vi "Interfaz_Computador.vi"() -> ()   [LabVIEW 2014]
uses:
  <vilib>/lvdsc/process/Deploy Library.vi
  <vilib>/lvdsc/process/Undeploy Library.vi
  <vilib>/lvdsc/NI_DSC.lvlib
panel:
  out "output cluster":T1
  out "error out":errorcluster
  in  "stop":bool
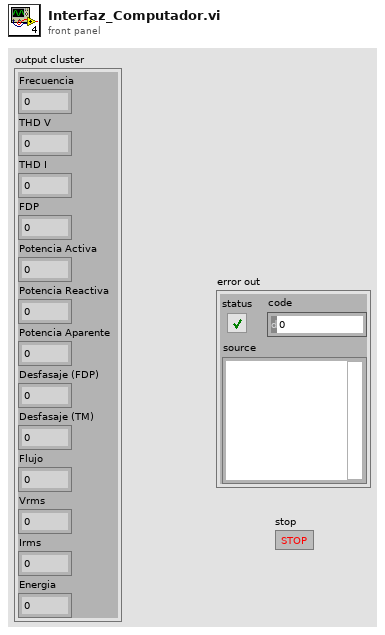
[diagram p1: front panel]
types:
  T1 = cluster{"Frecuencia":dbl, "THD V":dbl, "THD I":dbl, "FDP":dbl, "Potencia Activa":dbl, "Potencia Reactiva":dbl, "Potencia Aparente":dbl, "Desfasaje (FDP)":dbl, "Desfasaje (TM)":dbl, "Flujo":dbl, "Vrms":dbl, "Irms":dbl, "Energia":dbl}
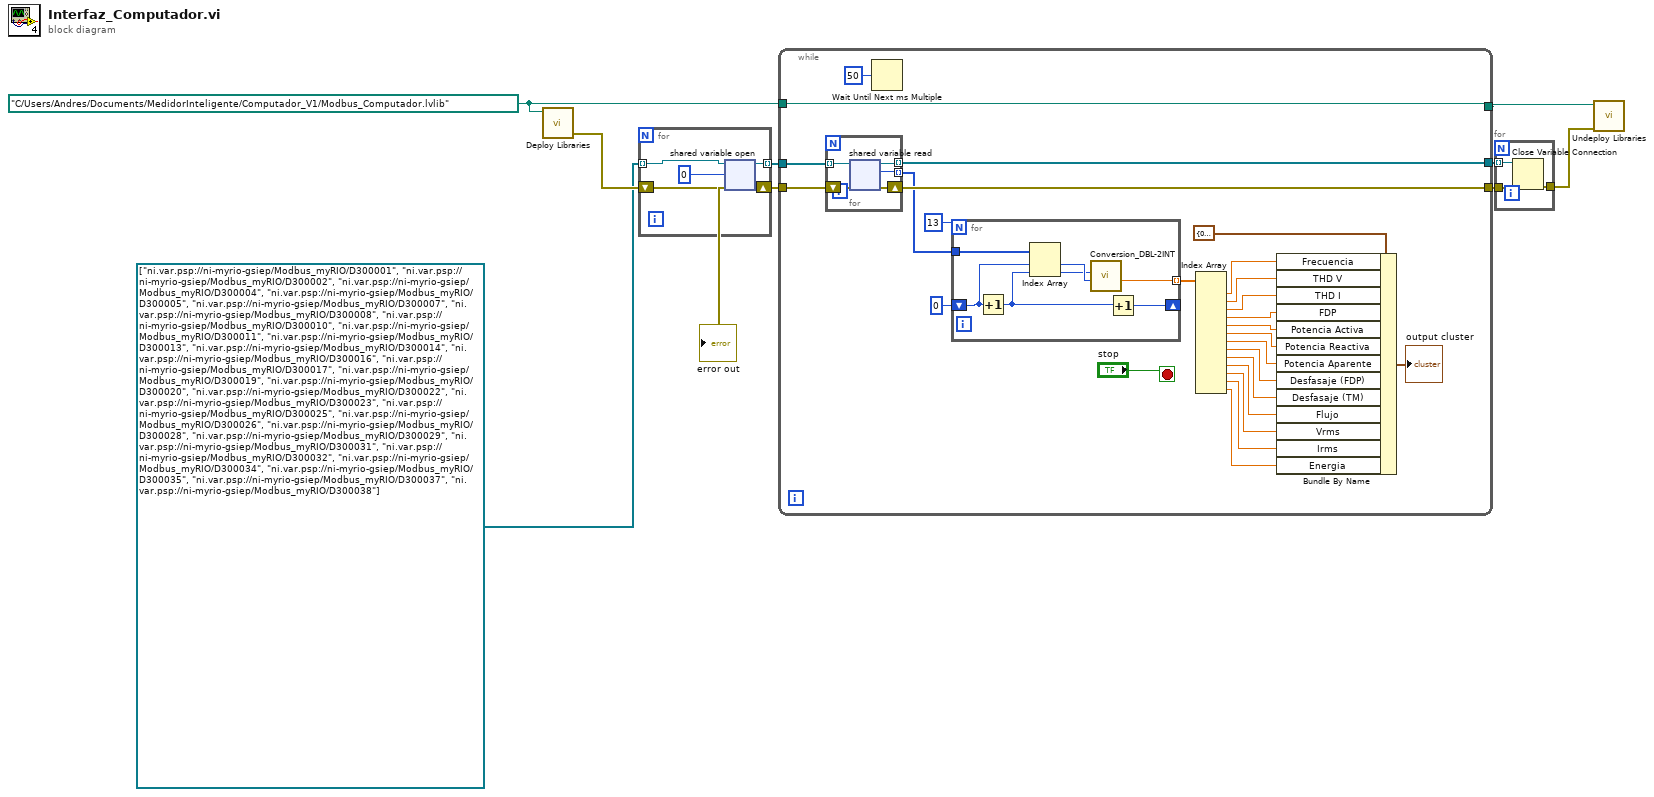
[diagram p0: block diagram]
diagram:
  w7 = path "C:/Users/Andres/Documents/MedidorInteligente/Computador_V1/Modbus_Computador.lvlib" ("library path")
  n1 = call-poly <vilib>:"Deploy Libraries.vi"("library path"=w7) -> ("error out"=w9:errorcluster)  [unwired: 8 in]
  n2 = for {
    tunnel: refnum<k21>[] ["ni.var.psp://ni-myrio-gsiep/Modbus_myRIO/D300001", "ni.var.psp://ni-myrio-gsiep/Modbus_myRIO/D300002", "ni.var.psp://ni-myrio-gsiep/Modbus_myRIO/D300004", "ni.var.psp://ni-myrio-gsiep/Modbus_myRIO/D300005", "ni.var.psp://ni-myrio-gsiep/Modbus_myRIO/D300007", "ni.var.psp://ni-myrio-gsiep/Modbus_myRIO/D300008", "ni.var.psp://ni-myrio-gsiep/Modbus_myRIO/D300010", "ni.var.psp://ni-myrio-gsiep/Modbus_myRIO/D300011", "ni.var.psp://ni-myrio-gsiep/Modbus_myRIO/D300013", "ni.var.psp://ni-myrio-gsiep/Modbus_myRIO/D300014", "ni.var.psp://ni-myrio-gsiep/Modbus_myRIO/D300016", "ni.var.psp://ni-myrio-gsiep/Modbus_myRIO/D300017", "ni.var.psp://ni-myrio-gsiep/Modbus_myRIO/D300019", "ni.var.psp://ni-myrio-gsiep/Modbus_myRIO/D300020", "ni.var.psp://ni-myrio-gsiep/Modbus_myRIO/D300022", "ni.var.psp://ni-myrio-gsiep/Modbus_myRIO/D300023", "ni.var.psp://ni-myrio-gsiep/Modbus_myRIO/D300025", "ni.var.psp://ni-myrio-gsiep/Modbus_myRIO/D300026", "ni.var.psp://ni-myrio-gsiep/Modbus_myRIO/D300028", "ni.var.psp://ni-myrio-gsiep/Modbus_myRIO/D300029", "ni.var.psp://ni-myrio-gsiep/Modbus_myRIO/D300031", "ni.var.psp://ni-myrio-gsiep/Modbus_myRIO/D300032", "ni.var.psp://ni-myrio-gsiep/Modbus_myRIO/D300034", "ni.var.psp://ni-myrio-gsiep/Modbus_myRIO/D300035", "ni.var.psp://ni-myrio-gsiep/Modbus_myRIO/D300037", "ni.var.psp://ni-myrio-gsiep/Modbus_myRIO/D300038"] -> [w10] mode=indexing
    shift-right: [w13] -> w8
    shift-left: w9 -> [w14]
    tunnel: [w12] -> w6 mode=indexing
    n3 = shared-variable-open(w10, w14, u32 0) -> (w12:refnum<k21>, w13:errorcluster)  [unwired: 1 in]
  }
  "error out" <- w8
  n4 = while {
    tunnel: w8 -> [w40]
    tunnel: [w39] -> w4
    tunnel: [w38] -> w5
    tunnel: w7 -> [w38]
    tunnel: w6 -> [w36]
    tunnel: [w34] -> w3
    stop <- "stop" stop-if-true
    n5 = for {
      tunnel: w36 -> [w50] mode=indexing
      shift-right: [w51] -> w39
      shift-left: w40 -> [w52]
      tunnel: [w49] -> w34 mode=indexing
      tunnel: [w48] -> w33 mode=indexing
      n6 = shared-variable-read(w50, w52) -> (w49:refnum<k21>, w51:errorcluster, w48:u32)  [unwired: 1 out]
    }
    n7 = Wait Until Next ms Multiple(millisecond multiple=u32 50) -> ()  [unwired: 1 out]
    n8 = for {
      N: 13 -> [_]
      tunnel: w33 -> [w47]
      shift-right: [w44] -> _
      shift-left: 0 -> [w46]
      tunnel: [w43] -> w29 mode=indexing
      n9 = Increment(x=w46) -> (x+1=w45:i32)
      n10 = Index Array(array=w47, index #1=w46, index #2=w45) -> (element #1=w42:u32, element #2=w41:u32)
      n11 = call "Conversion_DBL-2INT.vi"("Integer LOW"=w42, "Integer HIGH"=w41) -> ("Double"=w43:dbl)  [unwired: 2 in, 3 out]
      n12 = Increment(x=w45) -> (x+1=w44:i32)
    }
    n13 = Index Array(array=w29) -> (element #1=w28:dbl, element #2=w27:dbl, element #3=w26:dbl, element #4=w25:dbl, element #5=w24:dbl, element #6=w23:dbl, element #7=w22:dbl, element #8=w21:dbl, element #9=w20:dbl, element #10=w19:dbl, element #11=w18:dbl, element #12=w17:dbl, element #13=w16:dbl)  [unwired: 13 in]
    n14 = Bundle By Name(cluster=T1 {"Frecuencia"=0.0, "THD V"=0.0, "THD I"=0.0, "FDP"=0.0, "Potencia Activa"=0.0, "Potencia Reactiva"=0.0, "Potencia Aparente"=0.0, "Desfasaje (FDP)"=0.0, "Desfasaje (TM)"=0.0, "Flujo"=0.0, "Vrms"=0.0, "Irms"=0.0, "Energia"=0.0} ("output cluster"), "Frecuencia"=w28, "THD V"=w27, "THD I"=w26, "FDP"=w25, "Potencia Activa"=w24, "Potencia Reactiva"=w23, "Potencia Aparente"=w22, "Desfasaje (FDP)"=w21, "Desfasaje (TM)"=w20, "Flujo"=w19, "Vrms"=w18, "Irms"=w17, "Energia"=w16) -> (→"output cluster":T1)
  }
  n15 = for {
    tunnel: w4 -> [w55]
    tunnel: w3 -> [w54] mode=indexing
    tunnel: [w53] -> w2
    n16 = Close Variable Connection(8:w55, 11:w54) -> (0:w53:errorcluster)
  }
  n17 = call-poly <vilib>:"Undeploy Libraries.vi"("error in (no error)"=w2, "library path"=w5) -> ()  [unwired: 7 in, 1 out]
